vi "iTC-sample.vi"() -> ()   [LabVIEW 2014]
panel:
  in  "Seconds between \nMeasurements":dbl=5.0 min=0.0 max=9999999.0 step=1.0
  out "All Clear":bool
  out "Error":bool
  out "Run Start Time":string
  out "Last Measurement Taken":string
  out "Most Recent Error":string
  out "Heartbeat":bool
  in  "Heartbeat":bool
  in  "Temp Strip Chart":bool
  out "iTC Temperature Strip Chart":dynamicdata(graph)
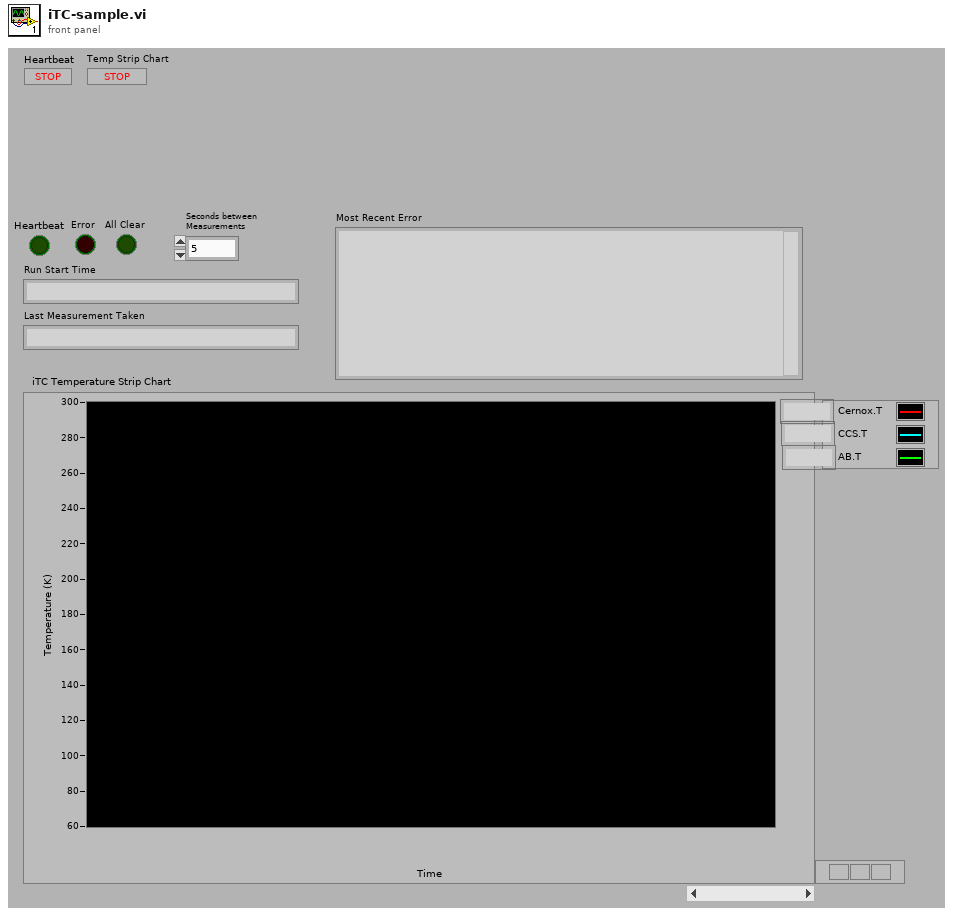
[diagram p1: front panel]
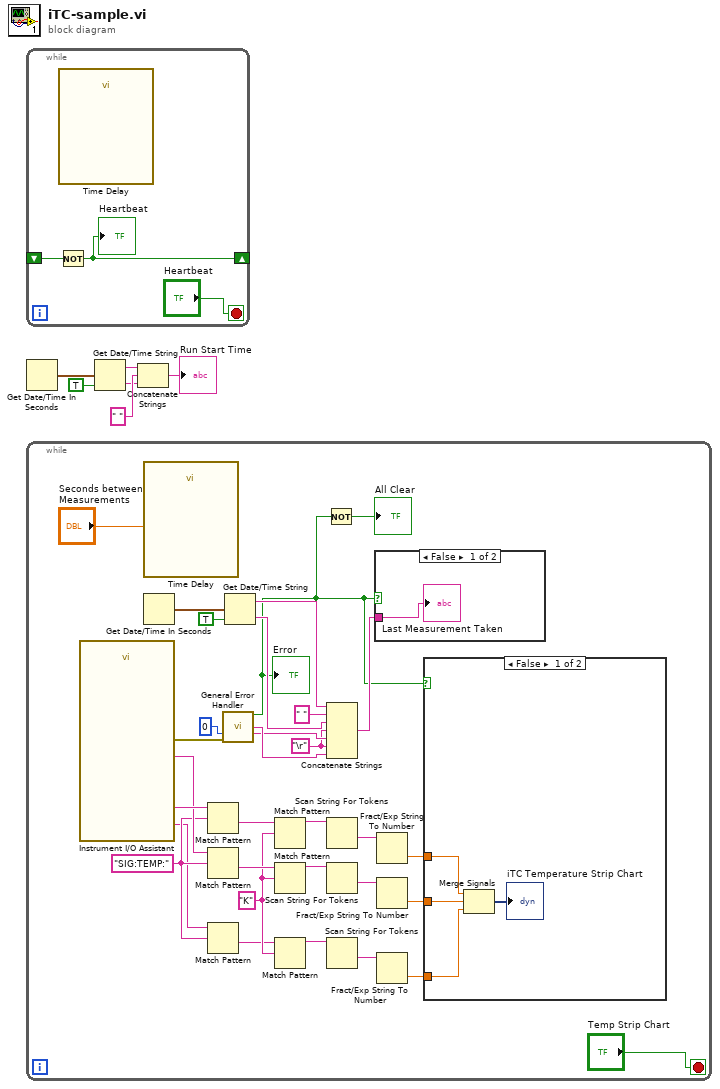
[diagram p0: block diagram]
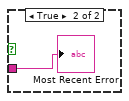
[diagram p3: hidden frame]
diagram:
  n1 = while {
    shift-right: [w7] -> _
    shift-left: _ -> [w9]
    stop <- "Heartbeat" stop-if-true
    n2 = Not(x=w9) -> (.not. x?=w7:bool)
    "Heartbeat" <- w7
    n3 = call "Time Delay"() -> ()  [unwired: 11 in, 1 out]
  }
  n4 = Get Date/Time In Seconds() -> (seconds since 1Jan1904=w5:timestamp)
  n5 = while {
    stop <- "Temp Strip Chart" stop-if-true
    w10 = "\r"
    w16 = "SIG:TEMP:"
    w15 = "K"
    n6 = call "Instrument I/O Assistant"() -> ("AB.T"=w14:string, "CCS.T"=w19:string, "Cernox.T"=w22:string, "error out"=w26:errorcluster)  [unwired: 23 in, 1 out]
    n7 = call "Time Delay"("Delay Time (s)"="Seconds between \nMeasurements") -> ()  [unwired: 10 in, 1 out]
    n8 = Get Date/Time In Seconds() -> (seconds since 1Jan1904=w37:timestamp)
    n9 = Match Pattern(string=w22, regular expression=w16) -> (after substring=w21:string)  [unwired: 1 in, 3 out]
    n10 = Match Pattern(string=w19, regular expression=w16) -> (after substring=w18:string)  [unwired: 1 in, 3 out]
    n11 = Match Pattern(string=w14, regular expression=w16) -> (after substring=w13:string)  [unwired: 1 in, 3 out]
    n12 = call <vilib>:"General Error Handler.vi"("type of dialog (OK msg:1)"=0, "error in (no error)"=w26) -> ("error?"=w24:bool, "source out"=w29:string, "message"=w28:string)  [unwired: 9 in, 2 out]
    "Error" <- w24
    n13 = Get Date/Time String(seconds (now)=w37, want seconds? (F)=TRUE) -> (date string=w35:string, time string=w33:string)  [unwired: 1 in]
    n14 = Match Pattern(string=w21, regular expression=w15) -> (before substring=w20:string)  [unwired: 1 in, 3 out]
    n15 = Match Pattern(string=w18, regular expression=w15) -> (before substring=w17:string)  [unwired: 1 in, 3 out]
    n16 = Match Pattern(string=w13, regular expression=w15) -> (before substring=w12:string)  [unwired: 1 in, 3 out]
    n17 = Not(x=w24) -> (.not. x?=→"All Clear":bool)
    n18 = Concatenate Strings(w35, " ", w33, w10, w28, w10, w29) -> (w27:string)
    n19 = Scan String For Tokens(9:w20) -> (1:w41:string)  [unwired: 5 in, 3 out]
    n20 = Scan String For Tokens(9:w17) -> (1:w39:string)  [unwired: 5 in, 3 out]
    n21 = Scan String For Tokens(9:w12) -> (1:w38:string)  [unwired: 5 in, 3 out]
    n22 = case shown="False" w24 {
      tunnel: w27 -> [w46 w47]
      frame False {
        "Last Measurement Taken" <- w46
      }
      frame True {
        "Most Recent Error" <- w47
      }
    }
    n23 = Fract/Exp String To Number(string=w41) -> (number=w32:dbl)  [unwired: 3 in, 1 out]
    n24 = Fract/Exp String To Number(string=w39) -> (number=w31:dbl)  [unwired: 3 in, 1 out]
    n25 = Fract/Exp String To Number(string=w38) -> (number=w30:dbl)  [unwired: 3 in, 1 out]
    n26 = case shown="False" w24 {
      tunnel: w32 -> [w44 _]
      tunnel: w31 -> [w43 _]
      tunnel: w30 -> [w42 _]
      frame False {
        n27 = Merge Signals(w44, w43, w42) -> (→"iTC Temperature Strip Chart":dynamicdata)
      }
      frame True {
      }
    }
  }
  n28 = Get Date/Time String(seconds (now)=w5, want seconds? (F)=TRUE) -> (date string=w4:string, time string=w2:string)  [unwired: 1 in]
  n29 = Concatenate Strings(w4, " ", w2) -> (→"Run Start Time":string)
